vi "Auto Align.vi"() -> (1 "y-axis":dbl, 2 "x-axis":dbl)   [LabVIEW 2012]
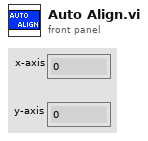
[diagram p1: front panel]
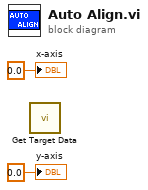
[diagram p0: block diagram]
diagram:
  n1 = call "Get Target Data.vi"() -> ()  [unwired: 12 in]
  "x-axis" <- 0.0 ("x-axis")
  "y-axis" <- 0.0 ("y-axis")
